vi "Fridge Turbo.vi"(7 "On OFF":bool, 8 "error in (no error)":errorcluster, 11 "IP Address in":string="128.174.164.8") -> (0 "error out":errorcluster)   [LabVIEW 2018]
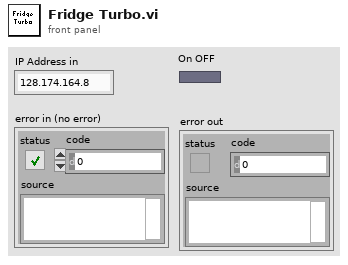
[diagram p1: front panel]
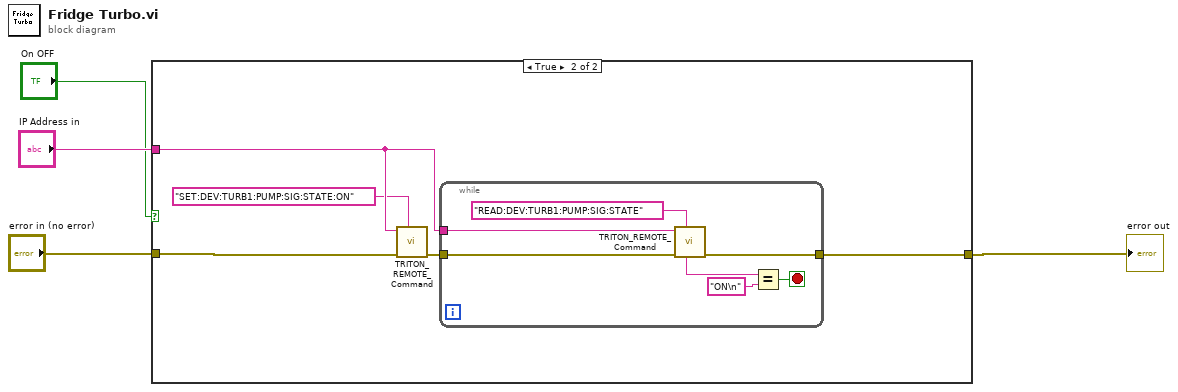
[diagram p0: block diagram]
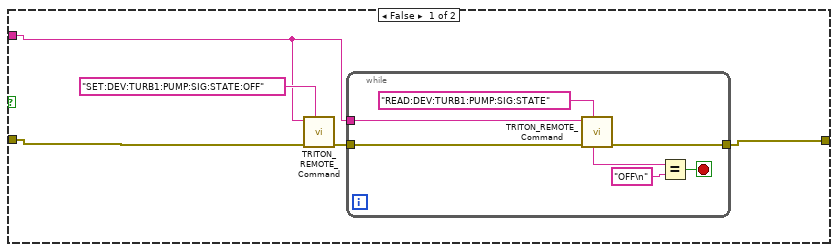
[diagram p2: hidden frame]
diagram:
  n1 = case shown="True" "On OFF" {
    tunnel: "IP Address in" -> [w5 w20]
    tunnel: "error in (no error)" -> [w6 w18]
    tunnel: [w7 w17] -> w2
    frame False {
      n2 = call "TRITON_REMOTE_Command.vi"("Command to send"="SET:DEV:TURB1:PUMP:SIG:STATE:OFF", "error in (no error)"=w6, "IP Address"=w5) -> ("error out"=w9:errorcluster)  [unwired: 6 in, 2 out]
      n3 = while {
        tunnel: w5 -> [w16]
        tunnel: w9 -> [w14]
        tunnel: [w10] -> w7
        stop <- w11 stop-if-true
        n4 = call "TRITON_REMOTE_Command.vi"("Command to send"="READ:DEV:TURB1:PUMP:SIG:STATE", "error in (no error)"=w14, "IP Address"=w16) -> ("error out"=w10:errorcluster, "Trimmed String"=w13:string)  [unwired: 6 in, 1 out]
        n5 = Equal?(x=w13, y="OFF\n") -> (x = y?=w11:bool)
      }
    }
    frame True {
      n6 = call "TRITON_REMOTE_Command.vi"("Command to send"="SET:DEV:TURB1:PUMP:SIG:STATE:ON", "error in (no error)"=w18, "IP Address"=w20) -> ("error out"=w21:errorcluster)  [unwired: 6 in, 2 out]
      n7 = while {
        tunnel: w20 -> [w28]
        tunnel: w21 -> [w26]
        tunnel: [w22] -> w17
        stop <- w23 stop-if-true
        n8 = call "TRITON_REMOTE_Command.vi"("Command to send"="READ:DEV:TURB1:PUMP:SIG:STATE", "error in (no error)"=w26, "IP Address"=w28) -> ("error out"=w22:errorcluster, "Trimmed String"=w25:string)  [unwired: 6 in, 1 out]
        n9 = Equal?(x=w25, y="ON\n") -> (x = y?=w23:bool)
      }
    }
  }
  "error out" <- w2
